vi "Init Hardware.vi"(8 "error in (no error)":errorcluster, 11 "Micron Hyperion Driver in":refnum<class "Micron Hyperion Driver.lvclass">) -> (0 "error out":errorcluster, 3 "Micron Hyperion Driver out":refnum<class "Micron Hyperion Driver.lvclass">)   [LabVIEW 2016, in "Micron Hyperion Driver.lvclass"]
uses:
  Micron Hyperion Driver.lvclass
  C:/GitHub/NHMFL_Core/Libraries/Instruments/Micron Optics/Micron Optics Driver/Micron Optics Driver.lvclass
  C:/GitHub/NHMFL_Core/Libraries/Instruments/Instrument Driver/Instrument Driver.lvclass
  hyperion library source/h.Library/DETECTION/h.DETECTION.PeakDetectionPreset.ctl
  Instrument Driver/Instrument Driver.lvclass/Instrument Driver.ctl
  Micron Optics Driver/Micron Optics Driver.lvclass/Micron Optics Driver.ctl
  Micron Optics Driver/Write Peaks buffer.vi
  Micron Optics Driver/Write Number of peaks.vi
  Instrument Driver/Read Cycle period.vi
  Micron Optics Driver/Read Timeout.vi
  Micron Optics Driver/Read Micron Configuration.vi
  hyperion library source/h.Library.lvlib
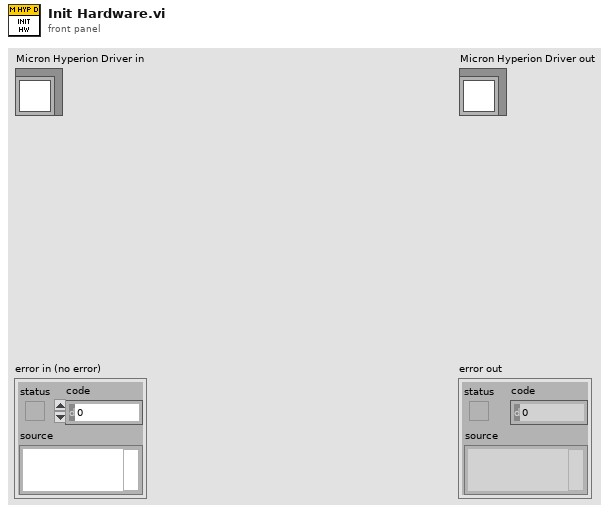
[diagram p1: front panel]
types:
  T1 = typedef "h.Library.lvlib/h.DETECTION.PeakDetectionPreset.ctl" = cluster{"Index":u8, "Name":string, "Description":string, "Detection Mode":enum32{"Valley", "Peak"}, "Averaging Window (pm)":i32, "Peak Width (pm)":i32, "Lockout Period (pm)":i32, "Search Window (ps)":i32, "Threshold Level":i32}
  T2 = typedef "Micron optics configuration.ctl" = cluster{"Reference channel":i32, "Detection Setting IDs":u8[], "Address":string, "Stream and average":bool}
  T3 = typedef "h.Library.lvlib/h.ACQ.PeaksData.ctl" = cluster{"SN":u64, "Time Stamp (ns)":u64, "Header Version":u16, "Peaks Wvls, nm":T4[]}
  T4 = typedef "h.Library.lvlib/h.ACQ.PeaksWvl.ctl" = cluster{"Peak Wvls, nm":dbl[]}
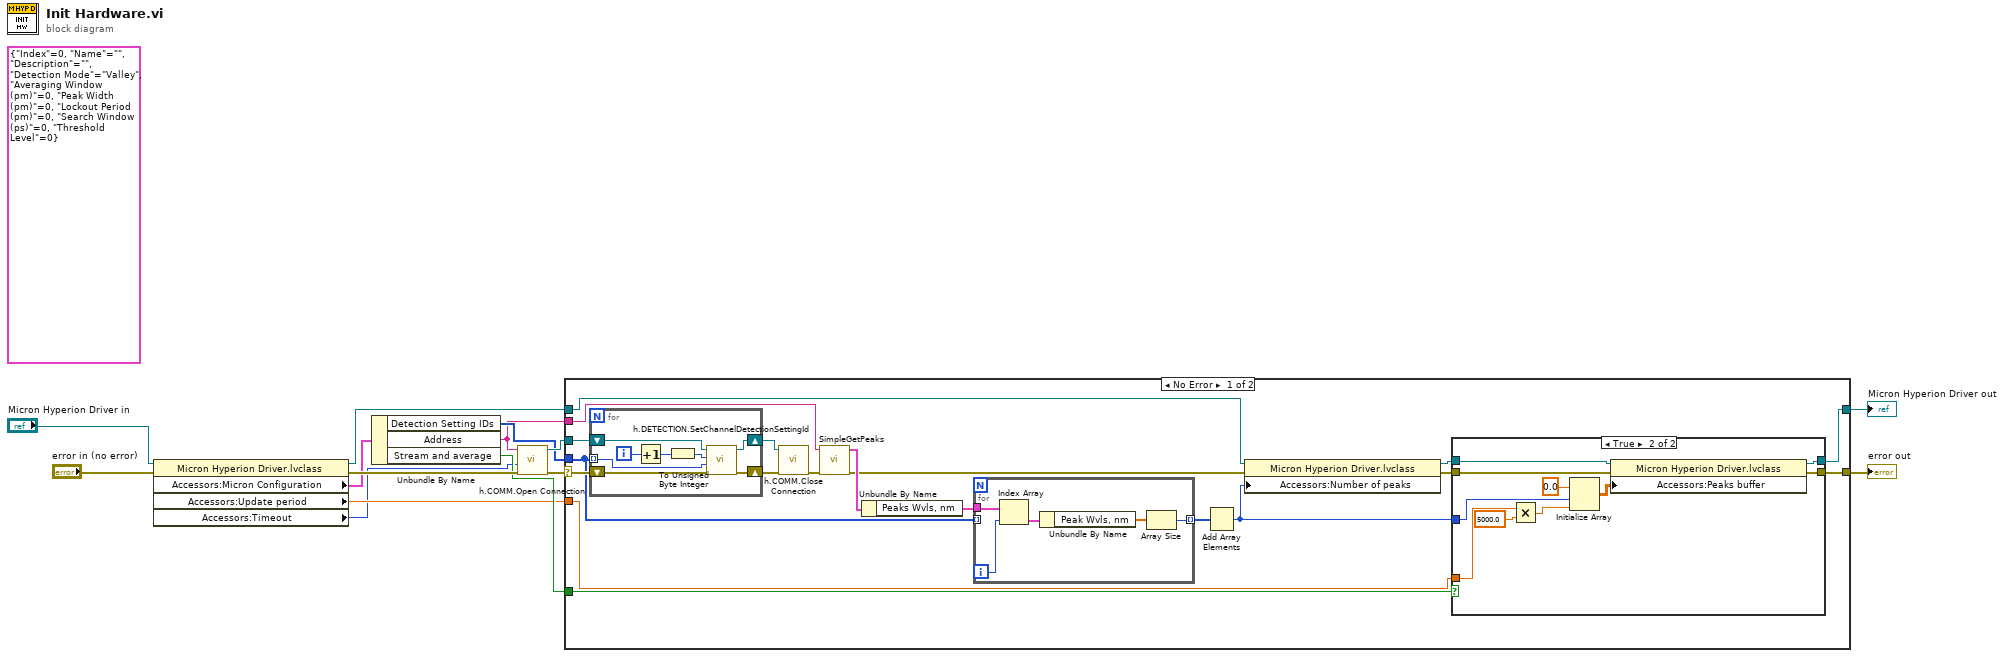
[diagram p0: block diagram]
diagram:
  (unwired) T1 {"Index"=0, "Name"="", "Description"="", "Detection Mode"=enum."Valley", "Averaging Window (pm)"=0, "Peak Width (pm)"=0, "Lockout Period (pm)"=0, "Search Window (ps)"=0, "Threshold Level"=0} ("Detection Setting")
  n1 = property class="Micron Hyperion Driver.lvclass"(reference="Micron Hyperion Driver in", error in="error in (no error)") -> (reference out=w2:refnum<class "Micron Hyperion Driver.lvclass">, error out=w13:errorcluster, "Accessors:Micron Configuration"=w10:T2, "Accessors:Update period"=w7:dbl, "Accessors:Timeout"=w4:i32)
  n2 = Unbundle By Name(w10) -> ("Detection Setting IDs"=w9:u8[], "Address"=w3:string, "Stream and average"=w8:bool)
  n3 = call "h.COMM.Open Connection.vi"("error in"=w13, "timeout (ms)"=w4, "Address"=w3) -> ("error out"=w1:errorcluster, "Connection ID"=w11:refnum<k5>)  [unwired: 7 in]
  n4 = case shown="No Error" w1 {
    selector: w1 -> [w17 w59]
    tunnel: w11 -> [w33 _]
    tunnel: w9 -> [w16 _]
    tunnel: w8 -> [w30 _]
    tunnel: w7 -> [w29 _]
    tunnel: [w28 w60] -> w6
    tunnel: [w27 w59] -> w5
    tunnel: w3 -> [w24 _]
    tunnel: w2 -> [w22 w60]
    frame No Error {
      n5 = for {
        tunnel: w16 -> [w43] mode=indexing
        shift-right: [w44] -> w31
        shift-left: w33 -> [w46]
        shift-right: [w45] -> w32
        shift-left: w17 -> [w42]
        i -> [w41]
        n6 = Increment(x=w41) -> (x+1=w40:i32)
        n7 = To Unsigned Byte Integer(number=w40) -> (unsigned 8bit integer=w39:u8)
        n8 = call "h.DETECTION.SetChannelDetectionSettingId.vi"("error in"=w42, "Detection Setting ID"=w43, "Channel Number"=w39, "Connection ID"=w46) -> ("error out"=w45:errorcluster, "Connection ID out"=w44:refnum<k5>)  [unwired: 6 in]
      }
      n9 = call "h.COMM.Close Connection.vi"("error in"=w32, "Connection ID"=w31) -> ("error out"=w23:errorcluster)  [unwired: 9 in]
      n10 = call "SimpleGetPeaks.vi"("Error In"=w23, "Address"=w24) -> ("Error Out"=w19:errorcluster, "Peaks Data"=w25:T3)  [unwired: 8 in]
      n11 = Unbundle By Name(w25) -> ("Peaks Wvls, nm"=w26:T4[])
      n12 = for {
        tunnel: w26 -> [w37]
        tunnel: [w35] -> w20 mode=indexing
        tunnel: w16 -> [_] mode=indexing
        i -> [w34]
        n13 = Index Array(array=w37, index=w34) -> (element=w38:T4)
        n14 = Unbundle By Name(w38) -> ("Peak Wvls, nm"=w36:dbl[])
        n15 = Array Size(array=w36) -> (size(s)=w35:i32)
      }
      n16 = Add Array Elements(numeric array=w20) -> (sum=w15:i32)
      n17 = property class="Micron Hyperion Driver.lvclass"(reference=w22, error in=w19, "Accessors:Number of peaks"=w15) -> (reference out=w21:refnum<class "Micron Hyperion Driver.lvclass">, error out=w18:errorcluster)
      n18 = case shown="True" w30 {
        tunnel: w21 -> [w47 w55]
        tunnel: w29 -> [_ w58]
        tunnel: w18 -> [w48 w53]
        tunnel: [w47 w52] -> w28
        tunnel: [w48 w51] -> w27
        tunnel: w15 -> [_ w49]
        frame False {
        }
        frame True {
          n19 = Multiply(x=w58, y=5000.0) -> (x*y=w50:dbl)
          n20 = Initialize Array(0.0, w49, w50) -> (w54:dbl[][])
          n21 = property class="Micron Hyperion Driver.lvclass"(reference=w55, error in=w53, "Accessors:Peaks buffer"=w54) -> (reference out=w52:refnum<class "Micron Hyperion Driver.lvclass">, error out=w51:errorcluster)
        }
      }
    }
    frame Error {
    }
  }
  "error out" <- w5
  "Micron Hyperion Driver out" <- w6
